vi "GetBedStatus.vi"(10 "url":string="http://192.168.0.112/") -> (2 "Vacant":bool=TRUE)   [LabVIEW 2015]
uses:
  <vilib>/httpClient/LabVIEWHTTPClient.lvlib
panel:
  in  "Ring 2":u16(ring)
  in  "Ring":u16(ring)
  out "after substring":string
  out "headers":string
  out "body":string
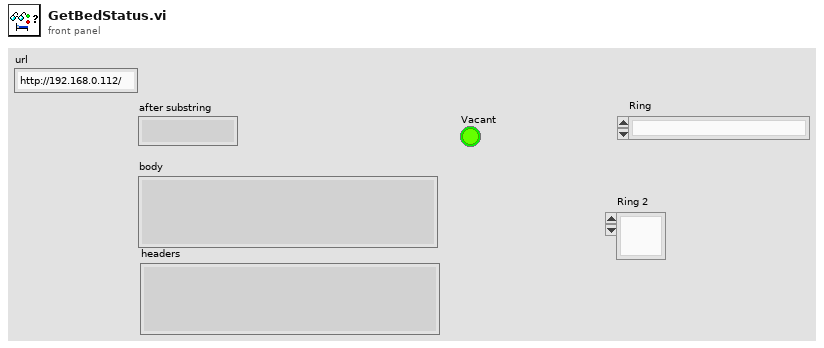
[diagram p1: front panel]
types:
  T1 = typedef "LabVIEWHTTPClient.lvlib/ClientHandle.ctl" = refnum<k1>
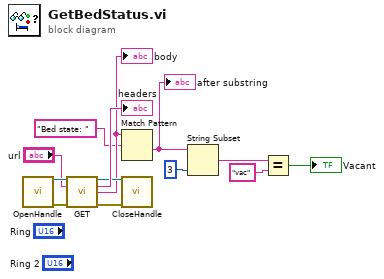
[diagram p0: block diagram]
diagram:
  n1 = call <vilib>:"OpenHandle.vi"() -> ("client handle out"=w13:T1, "error out"=w12:errorcluster)  [unwired: 14 in]
  n2 = call <vilib>:"GET.vi"("client handle"=w13, "url"="url", "error in (no error)"=w12) -> ("client handle out"=w9:T1, "headers"=→"headers":string, "body"=w7:string, "error out"=w8:errorcluster)  [unwired: 9 in]
  "body" <- w7
  n3 = Match Pattern(string=w7, regular expression="Bed state: ") -> (after substring=w5:string)  [unwired: 1 in, 3 out]
  "after substring" <- w5
  n4 = call <vilib>:"CloseHandle.vi"("client handle"=w9, "error in (no error)"=w8) -> ()  [unwired: 13 in, 1 out]
  n5 = String Subset(string=w5, length (rest)=3 ("length (rest)")) -> (substring=w3:string)  [unwired: 1 in]
  n6 = Equal?(x=w3, y="vac") -> (x = y?=→"Vacant":bool)
